vi "FrequencyResponse_v1.5.vi"() -> ()   [LabVIEW 2018]
uses:
  9a43e653-767e-4075-95b0-0c009614feea.vi
  25f52146-d521-482e-a5c2-4c0cf08532ff.vi
  6f2b9381-497d-4eca-9837-1c0e5003d3fc.vi
  d6a4aecf-3edc-4a6f-a0b4-04b53eacbead.vi
  bde50606-b3e8-4c81-9703-5e67d2be6f32.vi
panel:
  in  "Path":string="D:\\Users\\Stinky\\Documents\\FOMMC\\11.11.2020-20-200_data1\\"
  out "Min":dbl
  out "Sec":dbl
  out "H":dbl
  in  "Começar":bool
  out "Freq_Atual":dbl
  out "Tensão atual":dbl
  out "THD atual":dbl format="%.2p"
  in  "Diretorio final do arquivo":path=path "D:/Users/Stinky/Documents/FOMMC/11.11.2020-20-200_data1/data1.lvm" caption="Filename"
  in  "THD aceitavel":dbl=0.03 min=0.0 max=250.0
  in  "Gerador de Funções":refnum<visa-resource-name>="GPIB0::10::INSTR"
  in  "Osciloscópio*":refnum<visa-resource-name>="GPIB0::1::INSTR"
  in  "Tensão p/ causar Reentrância":dbl=0.2 min=0.0 max=250.0
  in  "Passo de Tensão (V)":dbl=0.05 min=0.0 max=250.0
  in  "Tensão SAT Fotodetector (V)":dbl=10.0 min=0.0 max=250.0
  in  "Passo Freq (Hz)":dbl=25.0 min=0.0 max=250.0
  in  "Freq Final (Hz)":dbl=5000.0 min=0.0 max=250.0
  in  "Freq Inicial (Hz)":dbl=500.0 min=0.0 max=250.0
  # "Endereços GPIB"
  # "Configurações Iniciais"
  # "*Canal 1: Sinal Interferométrico.\n Canal 2: Sinal do Gerador de Funções."
  # "Obs: Conectar Sync do GerFunc no \nTrigger Ext do osciloscópio."
  # "Tempo Decorrido"
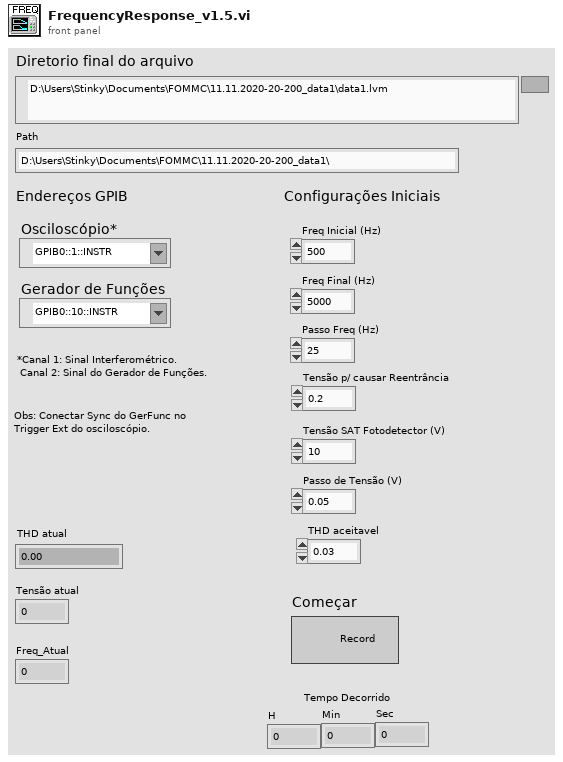
[diagram p1: front panel]
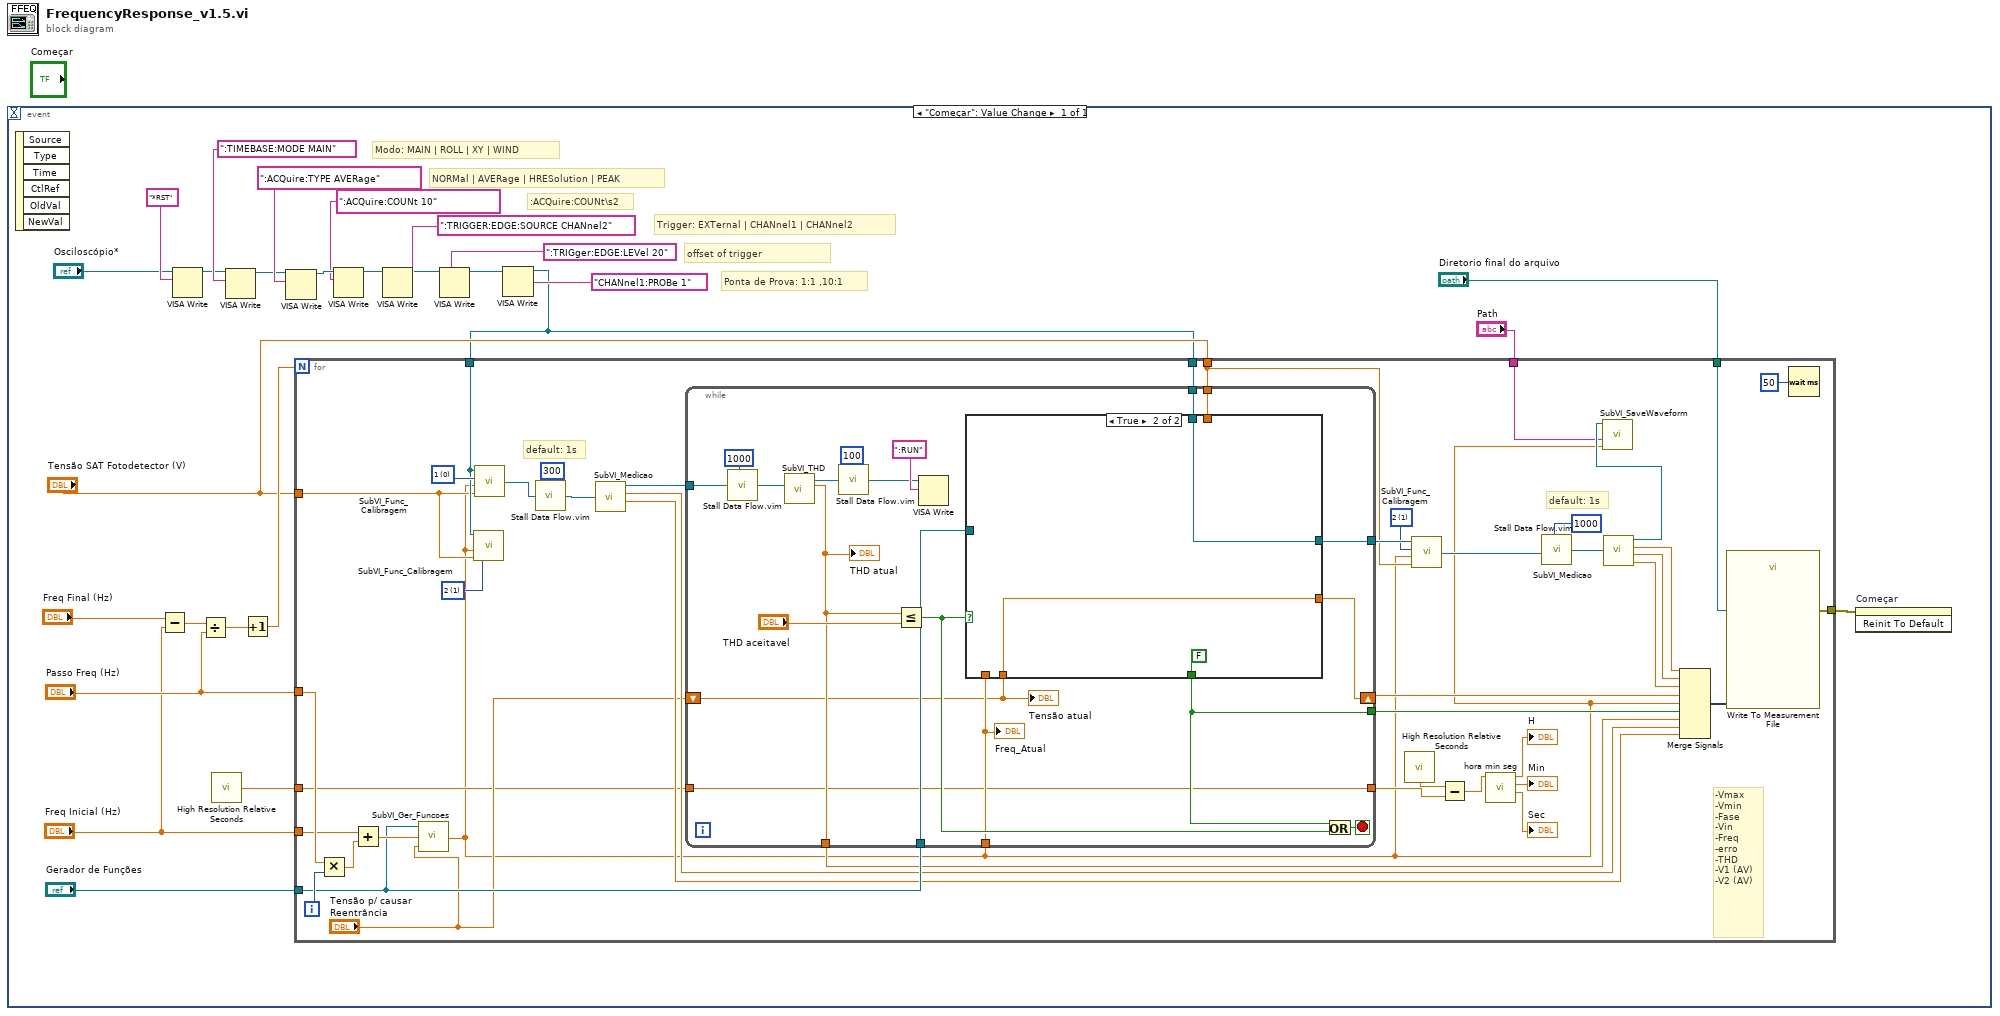
[diagram p0: block diagram]
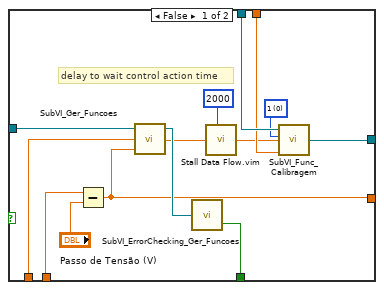
[diagram p2: hidden frame]
diagram:
  n1 = event shown="[0] \"Começar\": Value Change" {
    selector: _ -> [_]
    dyn-events: _ -> [_]
    timeout: _ -> [_]
    event "Começar": Value Change {
      # "offset of trigger"
      # ":ACQuire:COUNt\\s2"
      # "Trigger: EXTernal | CHANnel1 | CHANnel2"
      # "Ponta de Prova: 1:1 ,10:1"
      # "NORMal | AVERage | HRESolution | PEAK"
      # "Modo: MAIN | ROLL | XY | WIND"
      n2 = event-data() -> ()  [unwired: 1 in, 6 out]
      n3 = Subtract(x="Freq Final (Hz)", y="Freq Inicial (Hz)") -> (x-y=w20:dbl)
      n4 = VISA Write(VISA resource name="Osciloscópio*", write buffer="*RST") -> (VISA resource name out=w24:refnum<visa-resource-name>)  [unwired: 1 in, 2 out]
      n5 = Divide(x=w20, y="Passo Freq (Hz)") -> (x/y=w14:dbl)
      n6 = call <vilib>:"High Resolution Relative Seconds.vi"() -> ("relative seconds"=w9:dbl)
      n7 = VISA Write(VISA resource name=w24, write buffer=":TIMEBASE:MODE MAIN") -> (VISA resource name out=w22:refnum<visa-resource-name>)  [unwired: 1 in, 2 out]
      n8 = Increment(x=w14) -> (x+1=w19:dbl)
      n9 = VISA Write(VISA resource name=w22, write buffer=":ACQuire:TYPE AVERage") -> (VISA resource name out=w8:refnum<visa-resource-name>)  [unwired: 1 in, 2 out]
      n10 = VISA Write(VISA resource name=w8, write buffer=":ACQuire:COUNt 10") -> (VISA resource name out=w7:refnum<visa-resource-name>)  [unwired: 1 in, 2 out]
      n11 = VISA Write(VISA resource name=w7, write buffer=":TRIGGER:EDGE:SOURCE CHANnel2") -> (VISA resource name out=w5:refnum<visa-resource-name>)  [unwired: 1 in, 2 out]
      n12 = VISA Write(VISA resource name=w5, write buffer=":TRIGger:EDGE:LEVel 20") -> (VISA resource name out=w4:refnum<visa-resource-name>)  [unwired: 1 in, 2 out]
      n13 = VISA Write(VISA resource name=w4, write buffer="CHANnel1:PROBe 1") -> (VISA resource name out=w12:refnum<visa-resource-name>)  [unwired: 1 in, 2 out]
      n14 = for {
        N: w19 -> [_]
        tunnel: "Tensão SAT Fotodetector (V)" -> [w42]
        tunnel: "Passo Freq (Hz)" -> [w70]
        tunnel: "Gerador de Funções" -> [w66]
        tunnel: w12 -> [w44]
        tunnel: "Freq Inicial (Hz)" -> [w68]
        tunnel: "Tensão SAT Fotodetector (V)" -> [w56]
        tunnel: w12 -> [w65]
        tunnel: "Diretorio final do arquivo" -> [w31]
        tunnel: [w40] -> w10
        tunnel: w9 -> [w34]
        tunnel: "Path" -> [w29]
        i -> [w71]
        w43 = 1 items=["1", "2"] ("Canal")
        w57 = 1 items=["1", "2"] ("Canal")
        w59 = 0 items=["1", "2"] ("Canal")
        # "default: 1s"
        # "-Vmax\n-Vmin\n-Fase\n-Vin\n-Freq\n-erro\n-THD\n-V1 (AV)\n-V2 (AV)"
        # "default: 1s"
        n15 = Multiply(x=w70, y=w71) -> (x*y=w69:dbl)
        n16 = Add(x=w68, y=w69) -> (x+y=w67:dbl)
        n17 = call "SubVI_Ger_Funcoes.vi"("Tensão (Vp)"="Tensão p/ causar Reentrância", "Frequencia (Hz)"=w67, "Gerador de Funções"=w66) -> ("Freq_Atual"=w28:dbl)  [unwired: 2 out]
        n18 = call "SubVI_Func_Calibragem.vi"("Tensão SAT Fotodetector (V)"=w42, "Freq_atual"=w28, "Canal"=w43, "Osciloscópio"=w44) -> ()  [unwired: 1 out]
        n19 = call "SubVI_Func_Calibragem.vi"("Tensão SAT Fotodetector (V)"=w42, "Freq_atual"=w28, "Canal"=w59, "Osciloscópio"=w44) -> ("Osciloscópio out"=w47:refnum<visa-resource-name>)
        n20 = call "Stall Data Flow.vim"("value in"=w47, "milliseconds to wait"=u32 300) -> ("value out"=w46:refnum<visa-resource-name>)  [unwired: 1 out]
        n21 = call "SubVI_Medicao.vi"("Osciloscópio"=w46) -> ("Osciloscópio out"=w50:refnum<visa-resource-name>, "Vmax"=w49:dbl, "Vmin"=w48:dbl)  [unwired: 1 out]
        n22 = while {
          tunnel: w50 -> [w77]
          shift-right: [w90] -> w61
          shift-left: "Tensão p/ causar Reentrância" -> [w73]
          tunnel: w28 -> [w74]
          tunnel: w66 -> [w89]
          tunnel: w56 -> [w88]
          tunnel: w65 -> [w87]
          tunnel: [w85] -> w60
          tunnel: [w84] -> w58
          tunnel: [w75] -> w51
          tunnel: w34 -> [w72]
          tunnel: [w72] -> w33
          stop <- w86 stop-if-true
          n23 = call "Stall Data Flow.vim"("value in"=w77, "milliseconds to wait"=u32 1000) -> ("value out"=w83:refnum<visa-resource-name>)  [unwired: 1 out]
          n24 = call "SubVI_THD.vi"("Osciloscópio"=w83) -> ("THD"=w75:dbl, "VISA resource name out"=w80:refnum<visa-resource-name>)  [unwired: 9 in]
          "THD atual" <- w75
          n25 = call "Stall Data Flow.vim"("value in"=w80, "milliseconds to wait"=u32 100) -> ("value out"=w79:refnum<visa-resource-name>)  [unwired: 1 out]
          n26 = Less Or Equal?(x=w75, y="THD aceitavel") -> (x <= y?=w76:bool)
          n27 = VISA Write(VISA resource name=w79, write buffer=":RUN") -> ()  [unwired: 1 in, 3 out]
          n28 = case shown="True" w76 {
            tunnel: w73 -> [w105 w108]
            tunnel: [w92 w108] -> w90
            tunnel: w74 -> [w103 _]
            tunnel: w89 -> [w102 _]
            tunnel: w88 -> [w97 _]
            tunnel: w87 -> [w98 w106]
            tunnel: [w100 FALSE ("selection")] -> w85
            tunnel: [w99 w106] -> w84
            frame False {
              w96 = 0 items=["1", "2"] ("Canal")
              # "delay to wait control action time"
              n29 = Subtract(x=w105, y="Passo de Tensão (V)") -> (x-y=w92:dbl)
              n30 = call "SubVI_Ger_Funcoes.vi"("Tensão (Vp)"=w92, "Frequencia (Hz)"=w103, "Gerador de Funções"=w102) -> ("Freq_Atual"=w95:dbl, "VISA resource name out"=w101:refnum<visa-resource-name>)  [unwired: 1 out]
              n31 = call "SubVI_ErrorChecking_Ger_Funcoes.vi"("Gerador de Funções"=w101) -> ("ERROR"=w100:bool)  [unwired: 1 out]
              n32 = call "Stall Data Flow.vim"("value in"=w95, "milliseconds to wait"=u32 2000) -> ("value out"=w94:dbl)  [unwired: 1 out]
              n33 = call "SubVI_Func_Calibragem.vi"("Tensão SAT Fotodetector (V)"=w97, "Freq_atual"=w94, "Canal"=w96, "Osciloscópio"=w98) -> ("Osciloscópio out"=w99:refnum<visa-resource-name>)
            }
            frame True {
            }
          }
          n34 = Or(x=w85, y=w76) -> (x .or. y?=w86:bool)
          "Freq_Atual" <- w74
          "Tensão atual" <- w73
        }
        n35 = call <vilib>:"High Resolution Relative Seconds.vi"() -> ("relative seconds"=w38:dbl)
        n36 = call "SubVI_Func_Calibragem.vi"("Tensão SAT Fotodetector (V)"=w56, "Freq_atual"=w28, "Canal"=w57, "Osciloscópio"=w58) -> ("Osciloscópio out"=w54:refnum<visa-resource-name>)
        n37 = Subtract(x=w38, y=w33) -> (x-y=w39:dbl)
        n38 = call "hora min seg.vi"("Total time in seconds"=w39) -> ("Sec"=→"Sec":dbl, "Min"=→"Min":dbl, "H"=→"H":dbl)  [unwired: 8 in]
        n39 = call "Stall Data Flow.vim"("value in"=w54, "milliseconds to wait"=u32 1000) -> ("value out"=w32:refnum<visa-resource-name>)  [unwired: 1 out]
        n40 = call "SubVI_Medicao.vi"("Osciloscópio"=w32) -> ("Osciloscópio out"=w30:refnum<visa-resource-name>, "Vmax"=w64:dbl, "Vmin"=w63:dbl, "Fase"=w62:dbl)
        n41 = call "SubVI_SaveWaveform.vi"("frequency"=w28, "Path"=w29, "VISA resource name"=w30) -> ()  [unwired: 8 in, 1 out]
        n42 = Merge Signals(w64, w63, w62, w61, w28, w60, w51, w49, w48) -> (w52:dynamicdata)
        n43 = call "Write To Measurement File"("Signals"=w52, "Filename"=w31) -> ("error out"=w40:errorcluster)  [unwired: 15 in, 2 out]
        n44 = Wait (ms)(milliseconds to wait=u32 50) -> ()  [unwired: 1 out]
      }
      n45 = invoke on="Começar" class="Bool" method="Reinit To Default"(error in=w10) -> ()  [unwired: 2 in, 3 out]
    }
  }
